vi "oax_Convert Speed Info.vi"(10 "sampling info":T1={"sampling frequency"=51200.0, "total duration [s]"=10.0} {"sampling frequency" format="%#_6p"}, 11 "signal rotating speed":u16(ring) items=["3000 RPM", "1000-6000 RPM", "6000-1000 RPM", "1000-6000-1000 RPM"]) -> (2 "time period":dbl[](array[numeric]), 3 "speed":dbl[](array[numeric]))   [LabVIEW 2017]
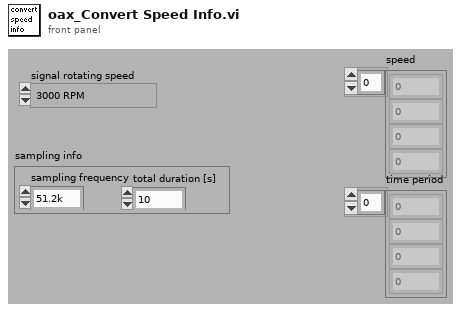
[diagram p1: front panel]
types:
  T1 = cluster{"sampling frequency":dbl, "total duration [s]":dbl}
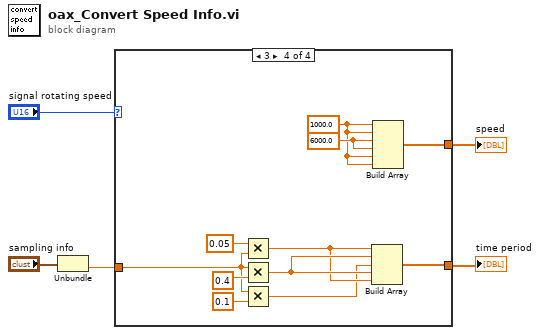
[diagram p0: block diagram]
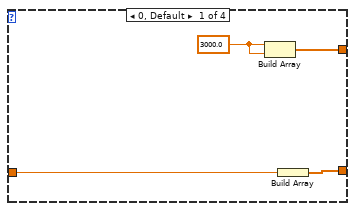
[diagram p2: hidden frame]
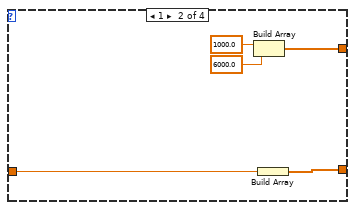
[diagram p3: hidden frame]
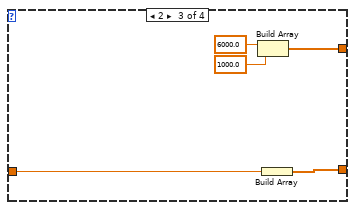
[diagram p4: hidden frame]
diagram:
  n1 = Unbundle("sampling info") -> ("total duration [s]"=w3:dbl)  [unwired: 1 out]
  n2 = case shown="3" "signal rotating speed" {
    tunnel: w3 -> [w8 w11 w16 w22]
    tunnel: [w7 w10 w17 w27] -> w2
    tunnel: [w9 w12 w15 w28] -> w1
    frame 0, Default {
      w6 = 3000.0
      n3 = Build Array(w6, w6) -> (w9:dbl[])
      n4 = Build Array(w8) -> (w7:dbl[])
    }
    frame 1 {
      n5 = Build Array(1000.0, 6000.0) -> (w12:dbl[])
      n6 = Build Array(w11) -> (w10:dbl[])
    }
    frame 2 {
      n7 = Build Array(6000.0, 1000.0) -> (w15:dbl[])
      n8 = Build Array(w16) -> (w17:dbl[])
    }
    frame 3 {
      w30 = 6000.0
      w29 = 1000.0
      n9 = Multiply(x=0.05, y=w22) -> (x*y=w24:dbl)
      n10 = Multiply(x=w22, y=0.4 ("x")) -> (x*y=w25:dbl)
      n11 = Multiply(x=w22, y=0.1) -> (x*y=w20:dbl)
      n12 = Build Array(w24, w25, w20, w25, w24) -> (w27:dbl[])
      n13 = Build Array(w29, w29, w30, w30, w29, w29) -> (w28:dbl[])
    }
  }
  "speed" <- w1
  "time period" <- w2
